vi "write_temp_to_file_activity_26.vi"() -> ()   [LabVIEW 2025]
panel:
  out "Temperature Chart":dbl(graph)
  in  "Number of points":i32
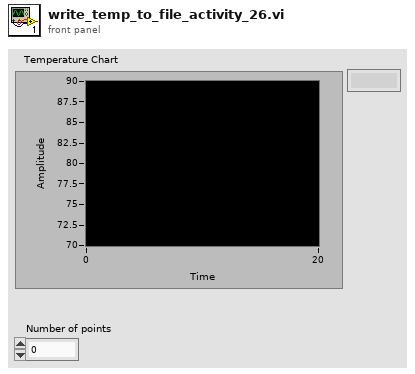
[diagram p1: front panel]
types:
  T1 = enum16{"open", "replace", "create", "open or create", "replace or create", "replace or create with confirmation"}
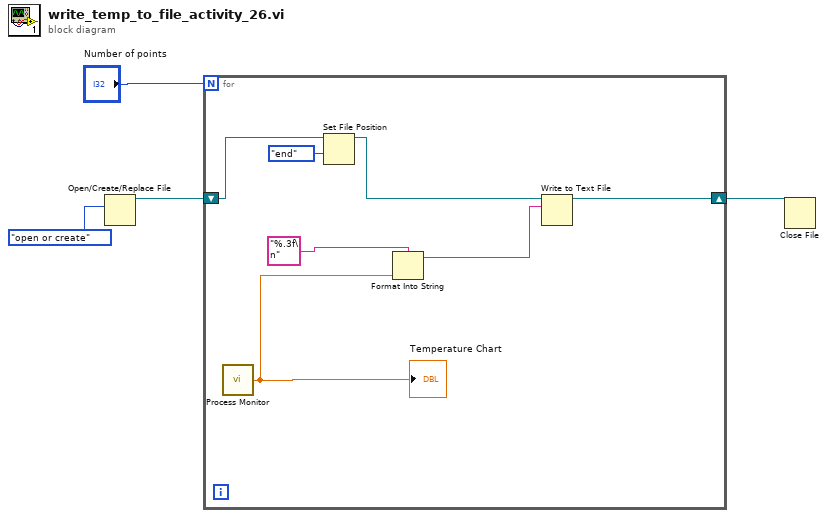
[diagram p0: block diagram]
diagram:
  n1 = Open/Create/Replace File(operation (0:open)=T1."open or create") -> (refnum out=w2:refnum<file>)  [unwired: 5 in, 2 out]
  n2 = for {
    N: "Number of points" -> [_]
    shift-right: [w5] -> w1
    shift-left: w2 -> [w7]
    n3 = call "Process Monitor.vi"() -> ("Temperature"=w9:dbl)  [unwired: 1 in, 2 out]
    "Temperature Chart" <- w9
    n4 = Set File Position(refnum=w7, from (0:start)=enum16{"start", "end", "current"}."end") -> (refnum out=w6:refnum<file>)  [unwired: 2 in, 1 out]
    n5 = Format Into String "Format Into String"(format string="%.3f\n", w9) -> (resulting string=w10:string)  [unwired: 2 in, 1 out]
    n6 = Write to Text File(file (use dialog)=w6, text=w10) -> (refnum out=w5:refnum<file>)  [unwired: 2 in, 2 out]
  }
  n7 = Close File(refnum=w1) -> ()  [unwired: 1 in, 2 out]
